vi "Telescope Home Focus.vi"(8 "error in (no error)":errorcluster, 11 "PRIME Telescope in":refnum<class "PRIME Telescope.lvclass">) -> (0 "error out":errorcluster, 3 "PRIME Telescope out":refnum<class "PRIME Telescope.lvclass">)   [LabVIEW 2024, in "PRIME Telescope.lvclass"]
uses:
  PRIME Telescope.lvclass
  PRIME Telescope.lvclass/PRIME Telescope.ctl
  Telescope.lvclass
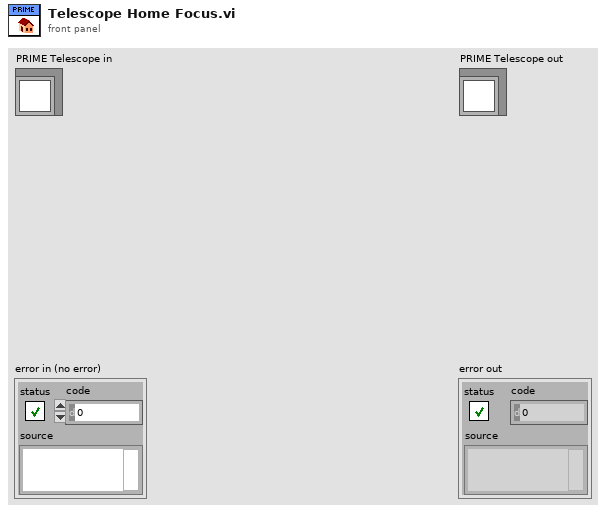
[diagram p1: front panel]
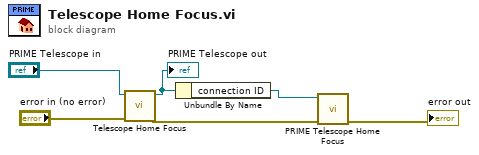
[diagram p0: block diagram]
diagram:
  n1 = call-parent "Telescope Home Focus.vi"("error in (no error)"="error in (no error)", "Telescope in"="PRIME Telescope in") -> ("error out"=w2:errorcluster, "Telescope out"=w4:refnum<class "PRIME Telescope.lvclass">)  [unwired: 8 in]
  "PRIME Telescope out" <- w4
  n2 = Unbundle By Name(w4) -> ("connection ID"=w3:refnum<k5>)
  n3 = call "PRIME Telescope Home Focus.vi"("error in (no error)"=w2, "connection ID"=w3) -> ("error out"=→"error out":errorcluster)  [unwired: 9 in]
